vi "RunTest.vi"(8 "error in (no error)":errorcluster, 11 "TestCaseMock in":refnum<class "TestCaseMock.lvclass">) -> (0 "error out":errorcluster, 3 "TestCaseMock out":refnum<class "TestCaseMock.lvclass">)   [LabVIEW 2019, in "TestSuiteTestSupport.lvlib" / "TestCaseMock.lvclass"]
doc: "Override to run the test and assert its state."
uses:
  TestCaseMock.lvclass
  TestCaseMock.lvclass/TestCaseMock.ctl
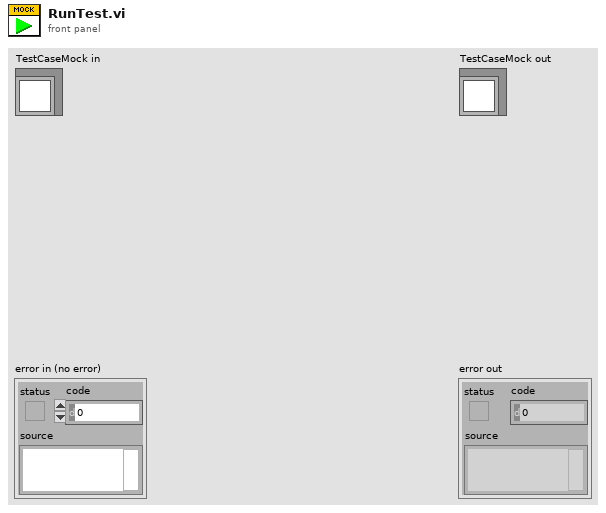
[diagram p1: front panel]
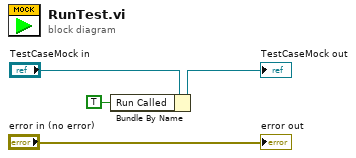
[diagram p0: block diagram]
diagram:
  n1 = Bundle By Name(cluster="TestCaseMock in", "Run Called"=TRUE) -> (→"TestCaseMock out":refnum<class "TestCaseMock.lvclass">)
  "error out" <- "error in (no error)"
